vi "IFD Merge.vi"(8 "error in (no error)":errorcluster, 10 "subIFD":refnum<class "IFD.lvclass">, 11 "main IFD":refnum<class "IFD.lvclass">) -> (0 "error out":errorcluster, 3 "IFD out":refnum<class "IFD.lvclass">)   [LabVIEW 2016, in "IFD.lvclass"]
uses:
  IFD.lvclass
  IFD.lvclass/IFD.ctl
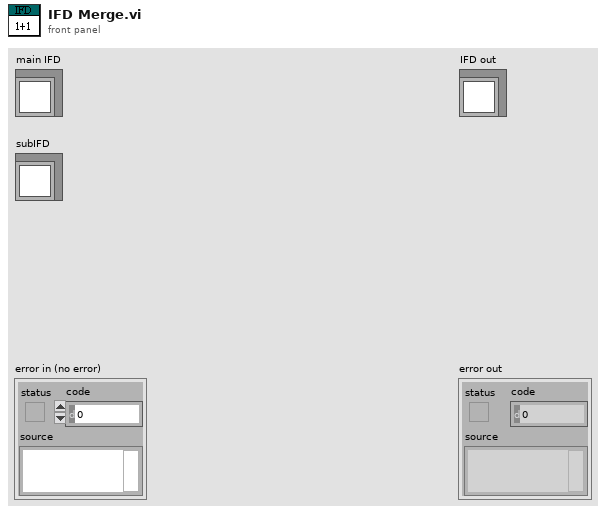
[diagram p1: front panel]
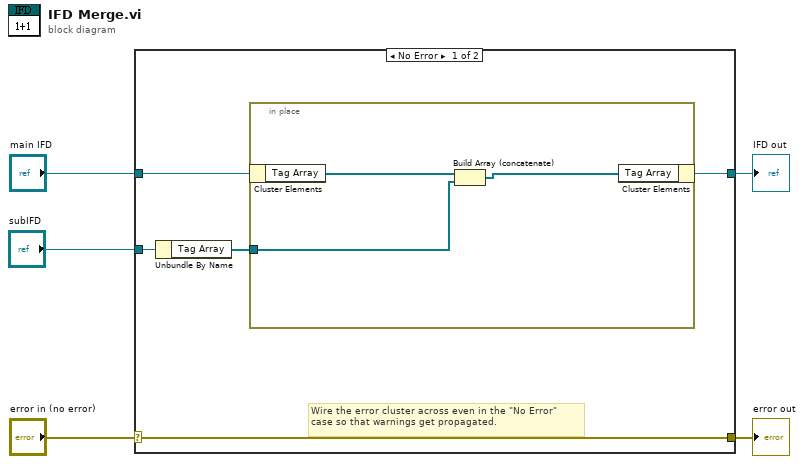
[diagram p0: block diagram]
diagram:
  n1 = case shown="No Error" "error in (no error)" {
    selector: "error in (no error)" -> [w10 w15]
    tunnel: [w10 w15] -> w4
    tunnel: [w6 w14] -> w2
    tunnel: "main IFD" -> [w9 w14]
    tunnel: "subIFD" -> [w8 _]
    frame No Error {
      # "Wire the error cluster across even in the \"No Error\"\ncase so that warnings get propagated."
      n2 = Unbundle By Name(w8) -> ("Tag Array"=w7:refnum<class "IFD_Tag.lvclass">[])
      n3 = in-place {
        in-place-border: w7 -> [w12]
        n4 = in-place-cluster #1(w9) -> ("Tag Array"=w13:refnum<class "IFD_Tag.lvclass">[])
        n5 = Build Array (concatenate)(w13, w12) -> (w11:refnum<class "IFD_Tag.lvclass">[])
        n6 = in-place-cluster #1("Tag Array"=w11) -> (w6:refnum<class "IFD.lvclass">)
      }
    }
    frame Error {
    }
  }
  "error out" <- w4
  "IFD out" <- w2
